vi "Run.vi"(8 "Error In":errorcluster, 10 "Tokens":refnum<class "Token.lvclass">[](array[class]), 11 "Parser In":refnum<class "Parser.lvclass">) -> (0 "Error Out":errorcluster, 2 "Abstract Syntax Tree":refnum<class "Root.lvclass">, 3 "Parser Out":refnum<class "Parser.lvclass">)   [LabVIEW 2018, in "Toolkit.lvlib" / "Parser.lvclass"]
uses:
  Parser.lvclass
  Nodes/Root/Root.lvclass
  Tokens/Token/Token.lvclass
  Parser.lvclass/Parser.ctl
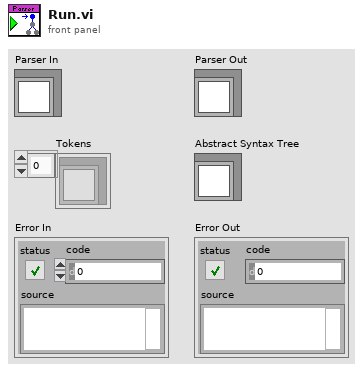
[diagram p1: front panel]
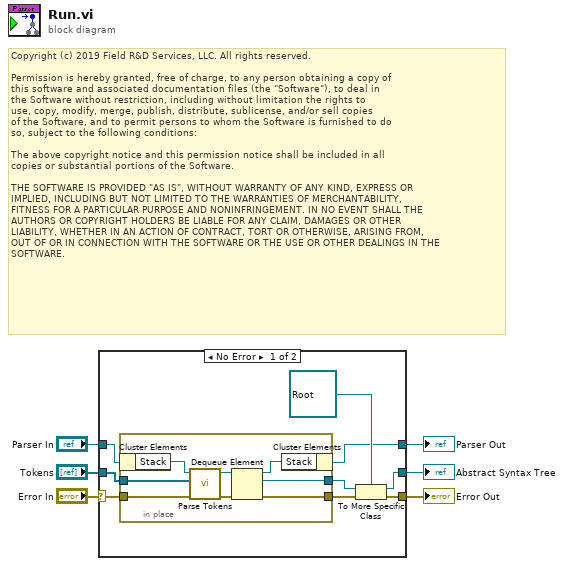
[diagram p0: block diagram]
diagram:
  # "Copyright (c) 2019 Field R&D Services, LLC. All rights reserved.\n\nPermission is hereby granted, free of charge, to any person obtaining a copy of\nthis software and associated documentation files (the \"Software\"), to deal in\nthe Software without restriction, including without limitation the rights to\nuse, copy, modify, merge, publish, distribute, sublicense, and/or sell copies\nof the Software, and to permit persons to whom the Software is furnished to do\nso, subject to the following conditions:\n\nThe above copyright notice and this permission notice shall be included in all\ncopies or substantial portions of the Software.\n\nTHE SOFTWARE IS PROVIDED \"AS IS\", WITHOUT WARRANTY OF ANY KIND, EXPRESS OR\nIMPLIED, INCLUDING BUT NOT LIMITED TO THE WARRANTIES OF MERCHANTABILITY,\nFITNESS FOR A PARTICULAR PURPOSE AND NONINFRINGEMENT. IN NO EVENT SHALL THE\nAUTHORS OR COPYRIGHT HOLDERS BE LIABLE FOR ANY CLAIM, DAMAGES OR OTHER\nLIABILITY, WHETHER IN AN ACTION OF CONTRACT, TORT OR OTHERWISE, ARISING FROM,\nOUT OF OR IN CONNECTION WITH THE SOFTWARE OR THE USE OR OTHER DEALINGS IN THE\nSOFTWARE."
  n1 = case shown="No Error" "Error In" {
    selector: "Error In" -> [w7 w25]
    tunnel: [w15 w25] -> w5
    tunnel: [w13 _] -> w4
    tunnel: "Tokens" -> [w12 _]
    tunnel: "Parser In" -> [w10 w24]
    tunnel: [w9 w24] -> w1
    frame No Error {
      n2 = in-place {
        in-place-border: w12 -> [w22]
        in-place-border: [w20] -> w11
        in-place-border: [w17] -> w8
        in-place-border: w7 -> [w16]
        n3 = in-place-cluster #1(w10) -> ("Stack"=w19:refnum<queue>)
        n4 = call "Parse Tokens.vi"("Error In"=w16, "Tokens"=w22, "Stack In"=w19) -> ("Error Out"=w23:errorcluster, "Stack Out"=w21:refnum<queue>)  [unwired: 7 in]
        n5 = Dequeue Element(queue=w21, error in (no error)=w23) -> (queue out=w18:refnum<queue>, element=w20:refnum<class "NonTerminal.lvclass">, error out=w17:errorcluster)  [unwired: 1 in, 1 out]
        n6 = in-place-cluster #1("Stack"=w18) -> (w9:refnum<class "Parser.lvclass">)
      }
      n7 = To More Specific Class(target class=refnum<class "Root.lvclass"> refnum ("Toolkit.lvlib:Nodes.lvlib:Root.lvclass"), reference=w11, error in=w8) -> (specific class reference=w13:refnum<class "Root.lvclass">, error out=w15:errorcluster)
    }
    frame Error {
    }
  }
  "Error Out" <- w5
  "Abstract Syntax Tree" <- w4
  "Parser Out" <- w1
